vi "Controller_Msgs.vi"() -> ()   [LabVIEW 2015]
uses:
  <userlib>/ROS for LabVIEW Software/ROS/Code/Console/Servers/ServerSubs/TopicDef.ctl
  <userlib>/ROS for LabVIEW Software/ROS/Code/SubVIs/_ROSDirection.ctl
  <vilib>/Platform/TimedLoop/XDataNode/timing_clust.ctl
  <vilib>/Platform/TimedLoop/XDataNode/nitl_modes.ctl
  <vilib>/Platform/TimedLoop/XDataNode/wakeup.ctl
  <userlib>/ROS for LabVIEW Software/ROS/MessageParsing/std_msgs/subs/parse_float64_scalar.vi
  <vilib>/FPGAPlugInAG/myRIO-1900/niLvFpga_Open_myRIO-1900.vi
  <vilib>/rvi/interface/common/dynamic/niFpgaDynamicAddResources.vi
  <vilib>/Utility/error.llb/Error Cluster From Error Code.vi
  <vilib>/rvi/errors/niLvFpgaAdjustHostInterfaceError.vi
  <vilib>/FPGAPlugInAG/Dynamic/niLvFpga_Close_Dynamic.vi
  <vilib>/rvi/interface/nirviOpenFPGA/nirviOpenFPGA.xnode
  FPGA Bitfiles/ViconProj_FPGATarget_CurrentControlle_AlrjX+GPFEk.lvbitx
  Current Controller.vi
  <vilib>/Platform/TimedLoop/XDataNode/XDataNode.xnode
  <vilib>/rvi/interface/nirviReadWriteControl/nirviReadWriteControl.xnode
  <vilib>/rvi/interface/nirviCloseFPGA/nirviCloseFPGA.xnode
  <vilib>/rvi/interface/Simulation/niFpgaSimulationCallBeginRW.vi
  NiFpgaLv.dll
  <vilib>/Platform/TimedLoop/XDataNode/XDNodeRunTimeDep.lvlib
panel:
  in  "Neunet Office":T1(tab)
  out "Control Signal":dbl(graph)
  in  "Definitions":T2={"Topic"="/controller", "Type"="std_msgs/Float64", "Action"=enum."Subscriber", "Update (ms)"=1, "queue size"=100}
  in  "Stop Button":bool
  out "FPGA Overflow?":bool
  out "error out":errorcluster
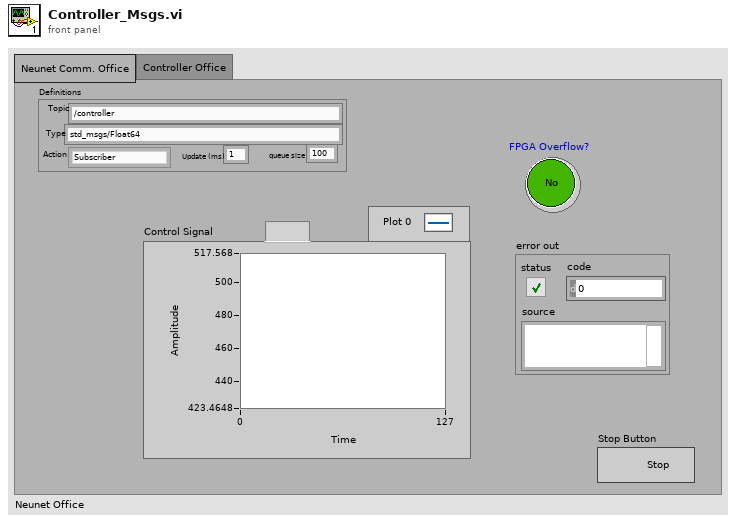
[diagram p1: front panel]
types:
  T1 = enum32{"Neunet Comm. Office", "Controller Office"}
  T2 = typedef "TopicDef.ctl" = cluster{"Topic":string, "Type":string, "Action":T3, "Update (ms)":u16, "queue size":u16}
  T3 = typedef "_ROSDirection.ctl" = enum16{"Node", "Publisher", "Subscriber", "ServiceClient", "ServiceProvider"}
  T4 = typedef "_ROSControl.ctl" = cluster{"topic port":u16, "Node":string, "topic":string, "type":string, "node port":u16, "error ":errorcluster, "Direction":T3, "Update (ms)":u16, "FIFO size":u16}
  T5 = typedef "XDNodeRunTimeDep.lvlib/timing_clust.ctl" = cluster{"Expected End [f-1]":u64, "Actual End [f-1]":u64, "Finished Late? [f-1]":bool, "Expected End [i-1]":u64, "Actual End [i-1]":u64, "Finished Late? [i-1]":bool, "Expected Start [i]":u64, "Actual Start [i]":u64, "Expected Start [f]":u64, "Actual Start [f]":u64, "Source Name":string, "Structure Name":string, "Period":i64, "Deadline":i64, "Offset":i64, "Start":i64, "Priority":i32, "Timeout":i32, "Mode":T6, "Wakeup Reason":T7, "Error":errorcluster, "Source Type":string, "Secondary Source Type":string, "Global End Time":u64, "Global Start Time":u64, "Frame Duration":u64, "Iteration Duration":u64, "Assigned CPU":i32, "I/O Scan Engine Mode":u32}
  T6 = typedef "XDNodeRunTimeDep.lvlib/nitl_modes.ctl" = enum32{"No Change", "Process missed periods, maintain original phase", "Discard missed periods, maintain original phase", "Process missed periods, ignore original phase", "Discard missed periods, ignore original phase"}
  T7 = typedef "XDNodeRunTimeDep.lvlib/wakeup.ctl" = enum32{"Normal", "Aborted", "Asynchronous wakeup", "Timing source error", "Timed loop error", "Timeout"}
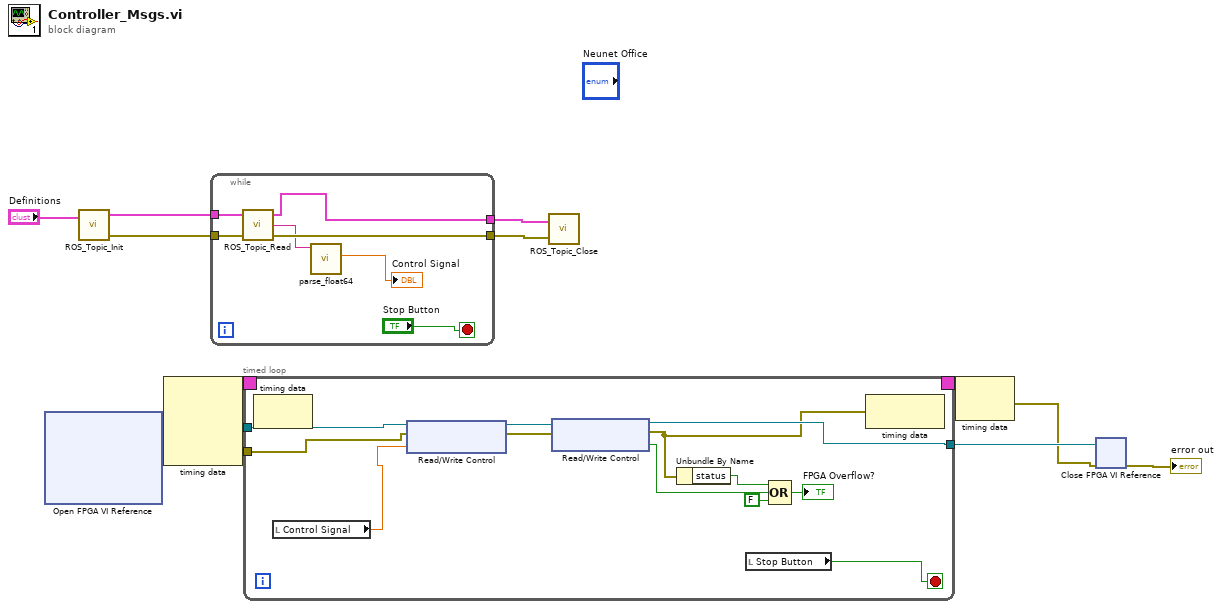
[diagram p0: block diagram]
diagram:
  n1 = xnode "Open FPGA VI Reference"() -> ("FPGA VI Reference Out"=w7:refnum<k20>, "error out"=w6:errorcluster)  [unwired: 2 in]
  n2 = call <userlib>:"ROS_Topic_Init.vi"("Definitions"="Definitions") -> ("ROS out"=w9:T4, "error out"=w8:errorcluster)  [unwired: 2 in]
  n3 = node-c288() -> (w5:T5)  [unwired: 4 in]
  n4 = while {
    tunnel: [w18] -> w12
    tunnel: [w15] -> w11
    tunnel: w9 -> [w16]
    tunnel: w8 -> [w17]
    stop <- "Stop Button" stop-if-true
    n5 = call <userlib>:"ROS_Topic_Read.vi"("error in (no error)"=w17, "ROS in"=w16) -> ("error out"=w15:errorcluster, "Reply"=w14:string, "ROS out"=w18:T4)  [unwired: 1 in]
    n6 = call-poly <userlib>:"parse_float64.vi"("msg in"=w14) -> ("number"=→"Control Signal":dbl)  [unwired: 4 in, 2 out]
  }
  n7 = timed-loop {
    timing: w5 -> [_]
    timing-out: [_] -> w4
    tunnel: w7 -> [w31]
    tunnel: w6 -> [w28]
    tunnel: [w21] -> w3
    stop <- w22 stop-if-true
    n8 = node-c288() -> ()  [unwired: 1 in, 1 out]
    n9 = local read "Control Signal"() -> (w29:dbl)
    n10 = xnode "Read/Write Control"("FPGA VI Reference In"=w31, "error in"=w28, "DAC Inlet Valve"=w29) -> ("FPGA VI Reference Out"=w30:refnum<k20>, "error out"=w27:errorcluster)
    n11 = xnode "Read/Write Control"("FPGA VI Reference In"=w30, "error in"=w27) -> ("FPGA VI Reference Out"=w21:refnum<k20>, "error out"=w20:errorcluster, "Inlet Overflow?"=w24:bool)
    n12 = Unbundle By Name(w20) -> ("status"=w26:bool)
    n13 = local read "Stop Button"() -> (w22:bool)
    n14 = Compound Arithmetic op=OR(w26, w24, FALSE ("value")) -> (→"FPGA Overflow?":bool)
    n15 = node-c288(w20) -> ()  [unwired: 1 out]
  }
  n16 = call <userlib>:"ROS_Topic_Close.vi"("error in"=w11, "ROS in"=w12) -> ()  [unwired: 2 in, 1 out]
  n17 = node-c288(w4) -> (w2:errorcluster)
  n18 = xnode "Close FPGA VI Reference"("FPGA VI Reference In"=w3, "error in"=w2) -> ("error out"=→"error out":errorcluster)
